vi "Get Water Level.vi"(8 "error in (no error)":cluster{"状态":bool, "代码":i32, "源":string} caption="错误输入（无错误）", 11 "水位输入":refnum<class "Water Level.lvclass">) -> (0 "error out":cluster{"状态":bool, "代码":i32, "源":string} caption="错误输出", 2 "水位":dbl)   [LabVIEW 2013, in "Water Level.lvlib" / "Water Level.lvclass"]
doc: "子类必须对该方法进行重写以返回水槽的水深。"
uses:
  Water Level.lvclass
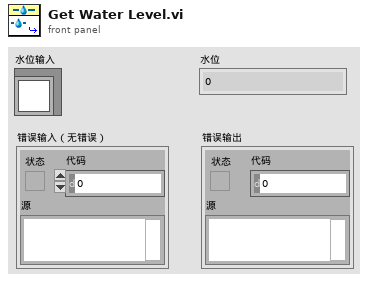
[diagram p1: front panel]
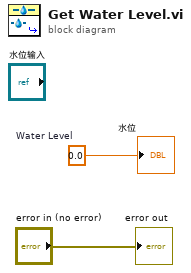
[diagram p0: block diagram]
diagram:
  w1 = 0.0  # Water Level
  "error out" <- "error in (no error)"
  "水位" <- w1
